vi "SaveSettingsAndCalibration.vi"(8 "error in (no error)":errorcluster, 11 "Cluster":T1={"Calibration Input"=[], "CalibrationResults"={"Center in Pixels"=[374.0120339529387, 375.46592887074246], "Angle"=0.022945275255000355, "Pixels/MHz X"=0.0, "Pixels/MHz Y"=0.0}, "Highlight"=[], "Running Script"=refnum}) -> (0 "error out":errorcluster)   [LabVIEW 2017]
uses:
  ExperimentVariables.ctl
  <vilib>/Utility/xml.llb/Write to XML File(string).vi
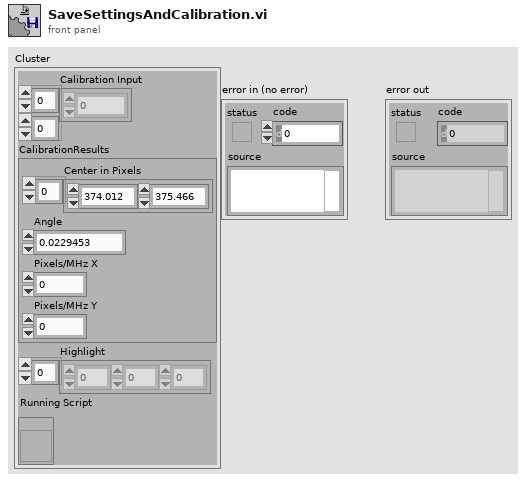
[diagram p1: front panel]
types:
  T1 = typedef "ExperimentVariables.ctl" = cluster{"Calibration Input":i32[][], "CalibrationResults":cluster{"Center in Pixels":dbl[], "Angle":dbl, "Pixels/MHz X":dbl, "Pixels/MHz Y":dbl}, "Highlight":i32[], "Running Script":refnum<vi>}
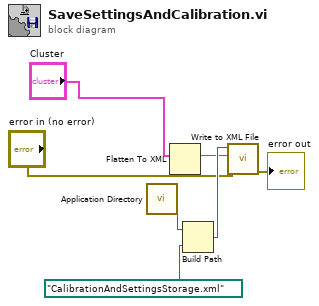
[diagram p0: block diagram]
diagram:
  n1 = call <vilib>:"Application Directory.vi"() -> ("Application Directory"=w5:path)
  n2 = Flatten To XML(anything="Cluster") -> (xml string=w4:string)
  n3 = Build Path(base path=w5, name or relative path=path "CalibrationAndSettingsStorage.xml" ("XML File Path")) -> (appended path=w7:path)
  n4 = call-poly <vilib>:"Write to XML File.vi"("error in (no error)"="error in (no error)", "XML Input"=w4, "XML File Path"=w7) -> ("error out"=→"error out":errorcluster)  [unwired: 6 in, 2 out]
